vi "aft_xmpl_Get_Initial_Coefficients.vi"(10 "unknown system coefficients":dbl[](array[numeric]), 11 "filter length":i32) -> (3 "initial coefficients":dbl[](array[numeric]))   [LabVIEW 2023]
doc: "Simulates the initial guess for the filter coefficients of the adaptive filter. This VI uses the unknown system coefficients plus noise as the initial guess."
uses:
  <vilib>/Analysis/NI_AALBase.lvlib
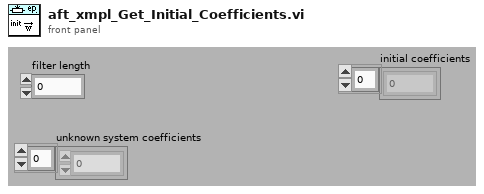
[diagram p1: front panel]
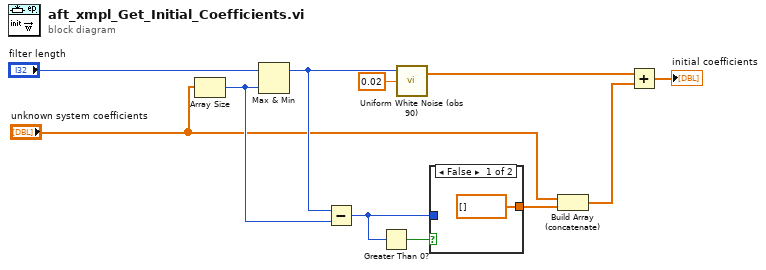
[diagram p0: block diagram]
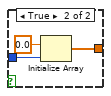
[diagram p2: hidden frame]
diagram:
  n1 = Array Size(array="unknown system coefficients") -> (size(s)=w7:i32)
  n2 = Max & Min(x="filter length", y=w7) -> (max(x,y)=w8:i32)  [unwired: 1 out]
  n3 = Subtract(x=w8, y=w7) -> (x-y=w5:i32)
  n4 = Greater Than 0?(x=w5) -> (x > 0?=w6:bool)
  n5 = call <vilib>:"Uniform White Noise (obs 90).vi"("amplitude"=0.02, "samples"=w8) -> ("uniform white noise"=w9:dbl[])  [unwired: 1 in, 1 out]
  n6 = case shown="False" w6 {
    tunnel: w5 -> [_ w15]
    tunnel: [dbl[] [] w13] -> w4
    frame False {
    }
    frame True {
      n7 = Initialize Array(0.0 ("element"), w15) -> (w13:dbl[])
    }
  }
  n8 = Build Array (concatenate)("unknown system coefficients", w4) -> (w2:dbl[])
  n9 = Add(x=w9, y=w2) -> (x+y=→"initial coefficients":dbl[])
